vi "0.0目標曲線計算.vi"(11 "mmin":T1={"Encoder  In"=[-14602.529690658634, -14602.529690658634, 14602.529690658634, 14602.529690658634], "RUN "=140.0, "MAX speed "=110.0, "累加AVSin "=[-300.0, 2.0, 139.49999999999977], "dt (s) in "=0.01, "START 減速"=FALSE}) -> (3 "mmout":T2)   [LabVIEW 2015]
panel:
  out "START 減速":bool
  out "dt (s) in":dbl=0.01 format="%#_13g"
  in  "累加AVSout":dbl[](array[numeric])
  out "累加AVSin":dbl[](array[numeric]) format="%#_13g"
  in  "Encoder Out":dbl[](array[numeric])
  in  "dt (s) out":dbl
  in  "做完了":bool
  out "MAX speed":dbl=90.0 format="%#_13g"
  out "RUN":dbl format="%#_13g"
  out "目標 Encoder In":dbl[](array[numeric])
  out "Current Speed":dbl=3.0
  out "Brake Distance":dbl=-0.0
  out "Distance Passed":dbl=399.21599999999523
  out "Distance Remain":dbl=0.03329555354736158
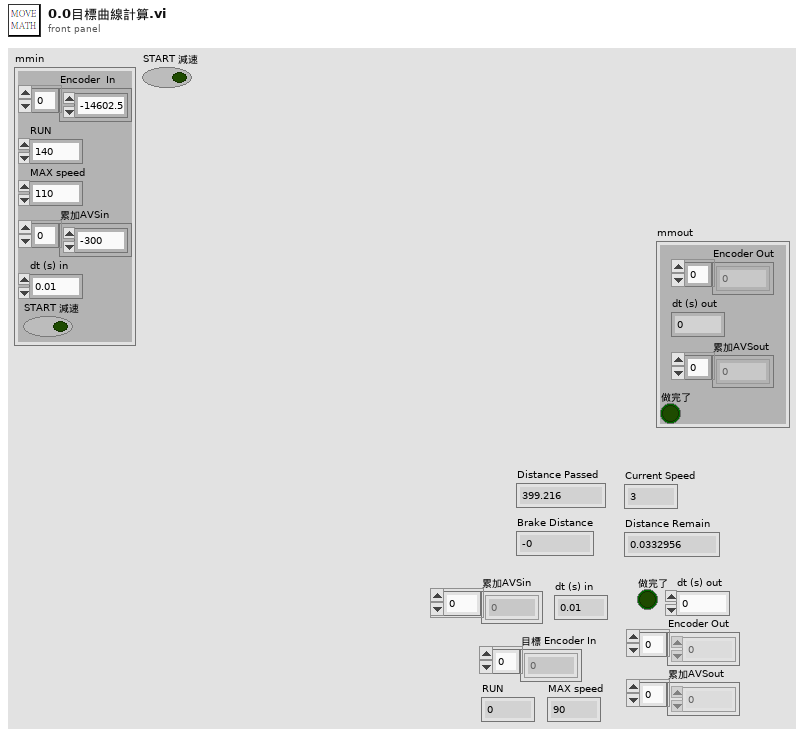
[diagram p1: front panel]
types:
  T1 = cluster{"Encoder  In":dbl[], "RUN ":dbl, "MAX speed ":dbl, "累加AVSin ":dbl[], "dt (s) in ":dbl, "START 減速":bool}
  T2 = cluster{"Encoder Out":dbl[], "dt (s) out ":dbl, "累加AVSout ":dbl[], "做完了 ":bool}
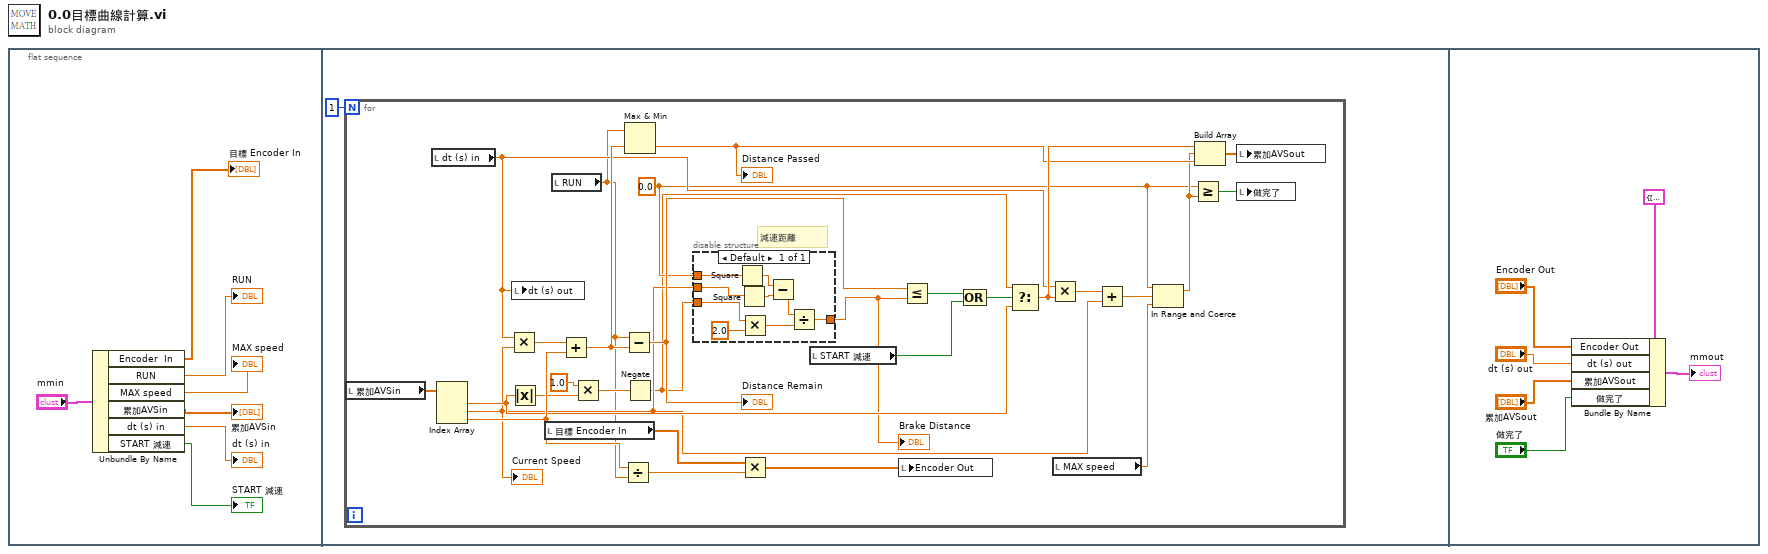
[diagram p0: block diagram]
diagram:
  n1 = flat-sequence {
    frame #0 {
      n2 = Unbundle By Name("mmin") -> ("Encoder  In"=→"目標 Encoder In":dbl[], "RUN"=→"RUN":dbl, "MAX speed"=→"MAX speed":dbl, "累加AVSin"=→"累加AVSin":dbl[], "dt (s) in"=→"dt (s) in":dbl, "START 減速"=→"START 減速":bool)
    }
    frame #1 {
      n3 = for {
        N: 1 -> [_]
        w13 = 0.0 ("累加AVSin")
        # "減速距離"
        n4 = local read "累加AVSin"() -> (w23:dbl[])
        n5 = local read "dt (s) in"() -> (w22:dbl)
        n6 = Index Array(array=w23) -> (element #1=w17:dbl, element #2=w12:dbl, element #3=w36:dbl)  [unwired: 3 in]
        "Current Speed" <- w12
        n7 = Multiply(x=w22, y=w12) -> (x*y=w33:dbl)
        n8 = Absolute Value(x=w17) -> (abs(x)=w18:dbl)
        n9 = local write "dt (s) out"(w22) -> ()
        n10 = local read "目標 Encoder In"() -> (w21:dbl[])
        n11 = local read "RUN"() -> (w9:dbl)
        n12 = Add(x=w33, y=w36) -> (x+y=w30:dbl)
        n13 = Multiply(x=1.0 ("(測試)減速放大倍率"), y=w18) -> (x*y=w27:dbl)
        n14 = Divide(x=w36, y=w9) -> (x/y=w32:dbl)
        n15 = Subtract(x=w9, y=w30) -> (x-y=w31:dbl)
        "Distance Remain" <- w31
        n16 = Max & Min(x=w9, y=w30) -> (min(x,y)=w25:dbl)  [unwired: 1 out]
        "Distance Passed" <- w25
        n17 = Negate(x=w27) -> (-x=w11:dbl)
        n18 = disable-structure shown="Default" {
          disable-tunnel: w13 -> [w46]
          disable-tunnel: w12 -> [w45]
          disable-tunnel: w11 -> [w42]
          disable-tunnel: [w38] -> w10
          frame Enabled {
            n19 = Square(x=w46) -> (x^2=w44:dbl)
            n20 = Square(x=w45) -> (x^2=w43:dbl)
            n21 = Multiply(x=w42, y=2.0) -> (x*y=w40:dbl)
            n22 = Subtract(x=w44, y=w43) -> (x-y=w39:dbl)
            n23 = Divide(x=w39, y=w40) -> (x/y=w38:dbl)
          }
        }
        "Brake Distance" <- w10
        n24 = Multiply(x=w21, y=w32) -> (x*y=w28:dbl[])
        n25 = local read "START 減速"() -> (w14:bool)
        n26 = local write "Encoder Out"(w28) -> ()
        n27 = Less Or Equal?(x=w31, y=w10) -> (x <= y?=w16:bool)
        n28 = Compound Arithmetic op=OR(w16, w14) -> (w15:bool)
        n29 = Select(t=w11, s=w15, f=w17) -> (s? t:f=w26:dbl)
        n30 = Multiply(x=w22, y=w26) -> (x*y=w34:dbl)
        n31 = local read "MAX speed"() -> (w24:dbl)
        n32 = Add(x=w34, y=w12) -> (x+y=w35:dbl)
        n33 = In Range and Coerce(upper limit=w13, x=w35, lower limit=w24) -> (coerced(x)=w19:dbl)  [unwired: 1 out]
        n34 = Greater Or Equal?(x=w13, y=w19) -> (x >= y?=w29:bool)
        n35 = Build Array(w26, w19, w25) -> (w20:dbl[])
        n36 = local write "累加AVSout"(w20) -> ()
        n37 = local write "做完了"(w29) -> ()
      }
    }
    frame #2 {
      n38 = Bundle By Name(cluster=T2 {"Encoder Out"=[0.0, 0.0, 0.0], "dt (s) out "=0.0, "累加AVSout "=[], "做完了 "=FALSE} ("input cluster"), "Encoder Out"="Encoder Out", "dt (s) out"="dt (s) out", "累加AVSout"="累加AVSout", "做完了"="做完了") -> (→"mmout":T2)
    }
  }
